vi "Test.vi"() -> ()   [LabVIEW 2020, in "RTAF.lvlib" / "Log.lvclass"]
uses:
  Log.lvclass
panel:
  out "Numeric":i32
  out "Period [ms]":u32
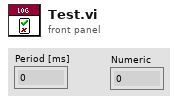
[diagram p1: front panel]
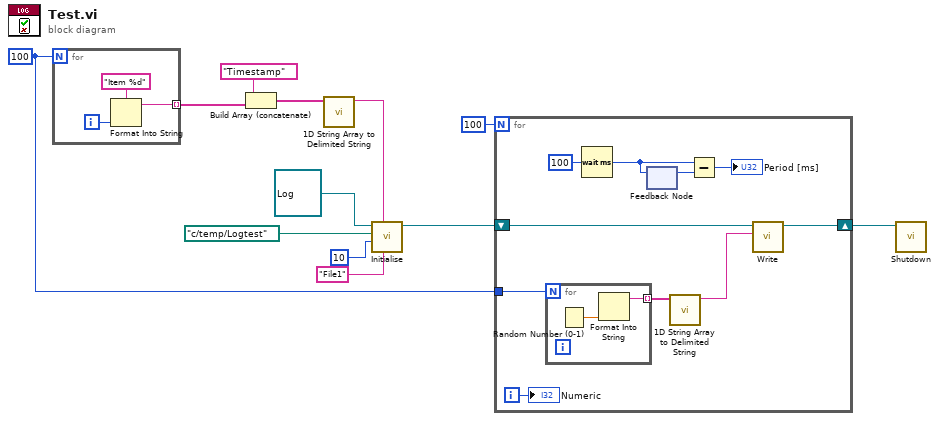
[diagram p0: block diagram]
diagram:
  w5 = 100
  n1 = for {
    N: w5 -> [_]
    tunnel: [w15] -> w9 mode=indexing
    i -> [w13]
    n2 = Format Into String(format string="Item %d", w13) -> (resulting string=w15:string)  [unwired: 2 in, 1 out]
  }
  n3 = Build Array (concatenate)("Timestamp" ("format string"), w9) -> (w2:string[])
  n4 = call <vilib>:"1D String Array to Delimited String.vi"("string array"=w2) -> ("delimited string"=w1:string)  [unwired: 10 in]
  n5 = call "Initialise.vi"("Filename"="File1", "Header"=w1, "Max Records"=10, "Directory"=path "c:/temp/Logtest", "Log in"=refnum<class "Log.lvclass"> refnum) -> ("Log out"=w12:refnum<class "Log.lvclass">)  [unwired: 5 in, 1 out]
  n6 = for {
    N: 100 -> [_]
    shift-right: [w24] -> w11
    shift-left: w12 -> [w25]
    tunnel: w5 -> [w18]
    i -> [w19]
    n7 = for {
      N: w18 -> [_]
      tunnel: [w26] -> w17 mode=indexing
      n8 = Random Number (0-1)() -> (number: 0 to 1=w27:dbl)
      n9 = Format Into String(w27) -> (resulting string=w26:string)  [unwired: 3 in, 1 out]
    }
    n10 = Wait (ms)(milliseconds to wait=u32 100) -> (millisecond timer value=w22:u32)
    n11 = feedback-in #1(w22) -> ()
    n12 = feedback #1() -> (w21:u32)  [unwired: 1 in]
    n13 = call <vilib>:"1D String Array to Delimited String.vi"("string array"=w17) -> ("delimited string"=w16:string)  [unwired: 10 in]
    n14 = Subtract(x=w22, y=w21) -> (x-y=→"Period [ms]":u32)
    n15 = call "Write.vi"("Message"=w16, "Log in"=w25) -> ("Log out"=w24:refnum<class "Log.lvclass">)  [unwired: 8 in, 1 out]
    "Numeric" <- w19
  }
  n16 = call "Shutdown.vi"("Log in"=w11) -> ()  [unwired: 10 in, 1 out]
